vi "Shutdown.vi"(8 "error in (no error)":errorcluster, 11 "PXImc Transceiver in":refnum<class "PXImc Transceiver.lvclass">) -> (0 "error out":errorcluster, 3 "PXImc Transceiver out":refnum<class "PXImc Transceiver.lvclass">)   [LabVIEW 2017, in "PXImc.lvlib" / "PXImc Transceiver.lvclass"]
uses:
  PXImc Transceiver.lvclass
  PXImc Transceiver.lvclass/PXImc Transceiver.ctl
  <vilib>/pximc/nipximc.lvlib
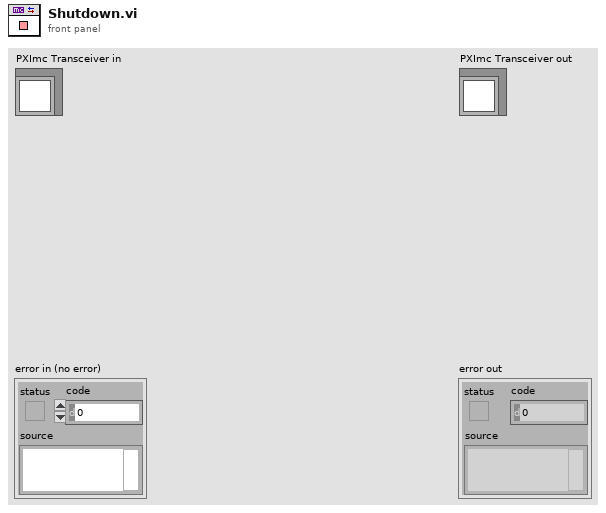
[diagram p1: front panel]
types:
  T1 = typedef "PXImc.lvlib/PXImc Transceiver.lvclass/PXImc Group Data.ctl" = cluster{"direction":T2, "transfers":T3[]}
  T2 = typedef "DSF Core.lvlibp/DSF Direction.ctl" = enum8{"Tx", "Rx"}
  T3 = typedef "PXImc.lvlib/PXImc Transceiver.lvclass/PXImc Transfer Data.ctl" = cluster{"stream id":u16, "session":refnum<k21>}
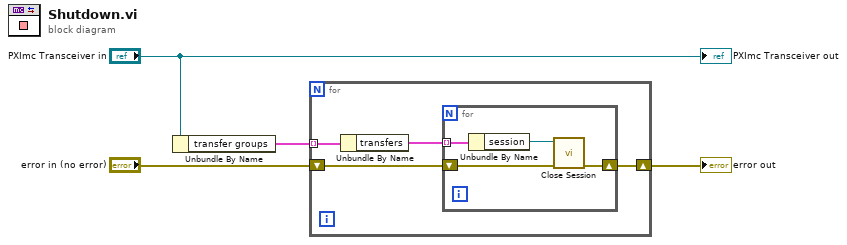
[diagram p0: block diagram]
diagram:
  n1 = Unbundle By Name("PXImc Transceiver in") -> ("transfer groups"=w3:T1[])
  n2 = for {
    tunnel: w3 -> [w8] mode=indexing
    shift-right: [w6] -> w1
    shift-left: "error in (no error)" -> [w5]
    n3 = Unbundle By Name(w8) -> ("transfers"=w7:T3[])
    n4 = for {
      tunnel: w7 -> [w12] mode=indexing
      shift-right: [w10] -> w6
      shift-left: w5 -> [w9]
      n5 = Unbundle By Name(w12) -> ("session"=w11:refnum<k21>)
      n6 = call <vilib>:"Close Session.vi"("error in (no error)"=w9, "session in"=w11) -> ("error out"=w10:errorcluster)  [unwired: 9 in]
    }
  }
  "error out" <- w1
  "PXImc Transceiver out" <- "PXImc Transceiver in"
